vi "Feedback 3 (SubVI).vi"(0 "reset_in":bool, 1 "eta_dot_last":dbl[](array[numeric]), 5 "Nu":dbl[](array[numeric]), 7 "Eta_last":dbl[](array[numeric]), 9 "Wait criteria":dbl[](array[numeric])=[2.0, 2.0, 2.0, 0.1], 11 "Restart criteria":dbl[](array[numeric])=[0.5, 0.5, 0.5, 0.1], 12 "Eta":dbl[](array[numeric]), 13 "Eta_d":dbl[](array[numeric]), 14 "Eta_ref":dbl[](array[numeric])) -> (4 "Boolean":bool, 6 "reset":bool, 8 "Eta_ref_out":dbl[](array[numeric]), 10 "u0":dbl[](array[numeric]), 15 "x0_out":dbl[](array[numeric]))   [LabVIEW 2011]
uses:
  <vilib>/imath/engines/lvmath2/RunTimeEngine/ErrorHandling/NIMS_Finalize Error.vi
  <vilib>/imath/engines/lvmath2/RunTimeEngine/Managers/WorkSpace/UID Generator.vi
  <vilib>/imath/engines/lvmath2/RunTimeEngine/RangeToken/NIMS_Range_R2 - Integer.vi
  <instcachedir>/0/NIMS_Range_R2 - Integer_8B99B1FAA0BB43C693F13B8216F464EC.lvgen/NIMS_Range_R2 - Integer_8B99B1FAA0BB43C693F13B8216F464EC_000.vi
  <vilib>/imath/engines/lvmath2/RunTimeEngine/Managers/SymbolTable/Clear UID.vi
  <vilib>/imath/engines/lvmath2/RunTimeEngine/NodeEndStatement/NIMS_NodeEndStatement_Output.vi
  <instcachedir>/0/NIMS_NodeEndStatement_Output_53EC0D466D134D7ABD903AC30B43404B.lvgen/NIMS_NodeEndStatement_Output_53EC0D466D134D7ABD903AC30B43404B_005.vi
  <vilib>/imath/engines/lvmath2/RunTimeEngine/CommandStatement/MC_CommandStatement_break.vi
  <vilib>/imath/engines/lvmath2/RunTimeEngine/VariableToken/Read/NIMS_Get Elements - RV(_) - Check.vi
  <instcachedir>/0/NIMS_Get Elements - RV(_) - Check_B511B9D8E05044FE80F9F088FE24B20C.lvgen/NIMS_Get Elements - RV(_) - Check_B511B9D8E05044FE80F9F088FE24B20C_000.vi
  <vilib>/imath/engines/lvmath2/RunTimeEngine/ErrorHandling/NIMS_Create Error From Enums.vi
  <vilib>/imath/engines/lvmath2/RunTimeEngine/ReplaceToken/NIMS_Replace - Check Linear.vi
  <instcachedir>/0/NIMS_Replace - Check Linear_276AD648BD064726893CCF9ED6E2A728.lvgen/NIMS_Replace - Check Linear_276AD648BD064726893CCF9ED6E2A728_001.vi
  <vilib>/imath/engines/lvmath2/RunTimeEngine/ReplaceToken/NIMS_Replace - Size Check _(_)=S.vi
  <instcachedir>/0/NIMS_Replace - Size Check _(_)=S_9ABE7AF2D26C43EAA05192D5C1E6C624.lvgen/NIMS_Replace - Size Check _(_)=S_9ABE7AF2D26C43EAA05192D5C1E6C624_000.vi
  <vilib>/imath/engines/lvmath2/RunTimeEngine/ReplaceToken/NIMS_Replace - V(S)=S.vi
  <instcachedir>/0/NIMS_Replace - V(S)=S_16B13A4565AB46F59881314645612498.lvgen/NIMS_Replace - V(S)=S_16B13A4565AB46F59881314645612498_000.vi
  <vilib>/imath/engines/lvmath2/RunTimeEngine/RunTimeType/NIMS_RunTimeType_From StrictType (excl LVString).vi
  <instcachedir>/0/NIMS_RunTimeType_From StrictType (excl LVString)_46AE8B54A11948F0BCCEB8091EE7AA4C.lvgen/NIMS_RunTimeType_From StrictType (excl LVString)_46AE8B54A11948F0BCCEB8091EE7AA4C_000.vi
  <vilib>/imath/engines/lvmath2/RunTimeEngine/LocalVariableDefStatement/MC_LocalVariableDefStatement_Display.vi
  <vilib>/imath/engines/lvmath2/RunTimeEngine/NodeEndStatement/NIMS_NodeEndStatement_Get Vector.vi
  <instcachedir>/0/NIMS_NodeEndStatement_Get Vector_50E2F48DC826428EA11CD85545CBACBE.lvgen/NIMS_NodeEndStatement_Get Vector_50E2F48DC826428EA11CD85545CBACBE_003.vi
  <instcachedir>/0/NIMS_NodeEndStatement_Get Vector_50E2F48DC826428EA11CD85545CBACBE.lvgen/NIMS_NodeEndStatement_Get Vector_50E2F48DC826428EA11CD85545CBACBE_001.vi
  <vilib>/imath/engines/lvmath/Functions/Error Handling/MergeErrorsWrapper.vi
  <instcachedir>/0/NIMS_NodeEndStatement_Output_53EC0D466D134D7ABD903AC30B43404B.lvgen/NIMS_NodeEndStatement_Output_53EC0D466D134D7ABD903AC30B43404B_013.vi
  <instcachedir>/0/NIMS_NodeEndStatement_Output_53EC0D466D134D7ABD903AC30B43404B.lvgen/NIMS_NodeEndStatement_Output_53EC0D466D134D7ABD903AC30B43404B_012.vi
  <instcachedir>/0/NIMS_NodeEndStatement_Output_53EC0D466D134D7ABD903AC30B43404B.lvgen/NIMS_NodeEndStatement_Output_53EC0D466D134D7ABD903AC30B43404B_001.vi
  <vilib>/imath/engines/lvmath2/RunTimeEngine/VariableToken/Read/NIMS_Get Elements - SorM(_) - Check.vi
  <instcachedir>/0/NIMS_Get Elements - SorM(_) - Check_6C920A4996D9400D8D9F035318A663F0.lvgen/NIMS_Get Elements - SorM(_) - Check_6C920A4996D9400D8D9F035318A663F0_007.vi
  <vilib>/imathl/engines/lvmath/Functions/Error Handling/Create Error.vi
  <instcachedir>/0/NIMS_Replace - Check Linear_276AD648BD064726893CCF9ED6E2A728.lvgen/NIMS_Replace - Check Linear_276AD648BD064726893CCF9ED6E2A728_006.vi
  <instcachedir>/0/NIMS_Replace - Size Check _(_)=S_9ABE7AF2D26C43EAA05192D5C1E6C624.lvgen/NIMS_Replace - Size Check _(_)=S_9ABE7AF2D26C43EAA05192D5C1E6C624_004.vi
  <vilib>/imath/engines/lvmath2/RunTimeEngine/ReplaceToken/NIMS_Replace - M(S)=S.vi
  <instcachedir>/0/NIMS_Replace - M(S)=S_FF4DE4724B384A588EB88F1DEAD450CF.lvgen/NIMS_Replace - M(S)=S_FF4DE4724B384A588EB88F1DEAD450CF_001.vi
  <vilib>/imath/engines/lvmath2/RunTimeEngine/ArithmeticOperatorToken/NIMS_ArithmeticOperator_multmx(M,CV).vi
  <instcachedir>/0/NIMS_ArithmeticOperator_multmx(M,CV)_B95E4EDD04E247939487CF1FF34819AA.lvgen/NIMS_ArithmeticOperator_multmx(M,CV)_B95E4EDD04E247939487CF1FF34819AA_000.vi
  <vilib>/imath/engines/lvmath2/RunTimeEngine/BuiltInFunctions/abs/NIMS_abs(signed).vi
  <instcachedir>/0/NIMS_abs(signed)_C4FCB8E6058B49B797C7C8D53CA5F6EC.lvgen/NIMS_abs(signed)_C4FCB8E6058B49B797C7C8D53CA5F6EC_000.vi
  <instcachedir>/0/NIMS_Get Elements - SorM(_) - Check_6C920A4996D9400D8D9F035318A663F0.lvgen/NIMS_Get Elements - SorM(_) - Check_6C920A4996D9400D8D9F035318A663F0_000.vi
  <vilib>/imath/engines/lvmath2/RunTimeEngine/ArithmeticOperatorToken/NIMS_ArithmeticOperator_minus.vi
  <instcachedir>/0/NIMS_ArithmeticOperator_minus_27860A2576AF4B729B9D72749D8AAD88.lvgen/NIMS_ArithmeticOperator_minus_27860A2576AF4B729B9D72749D8AAD88_003.vi
  <vilib>/imath/engines/lvmath2/RunTimeEngine/Managers/SymbolTable/NIMS_WorkSpace.lvlib
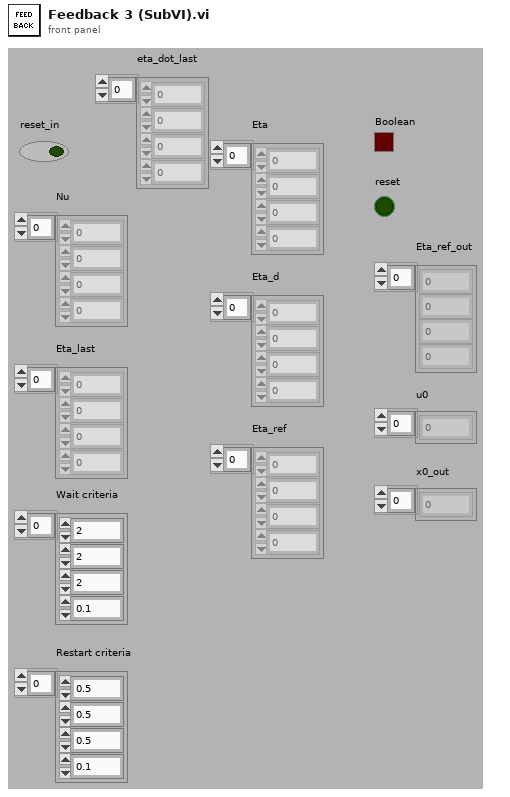
[diagram p1: front panel]
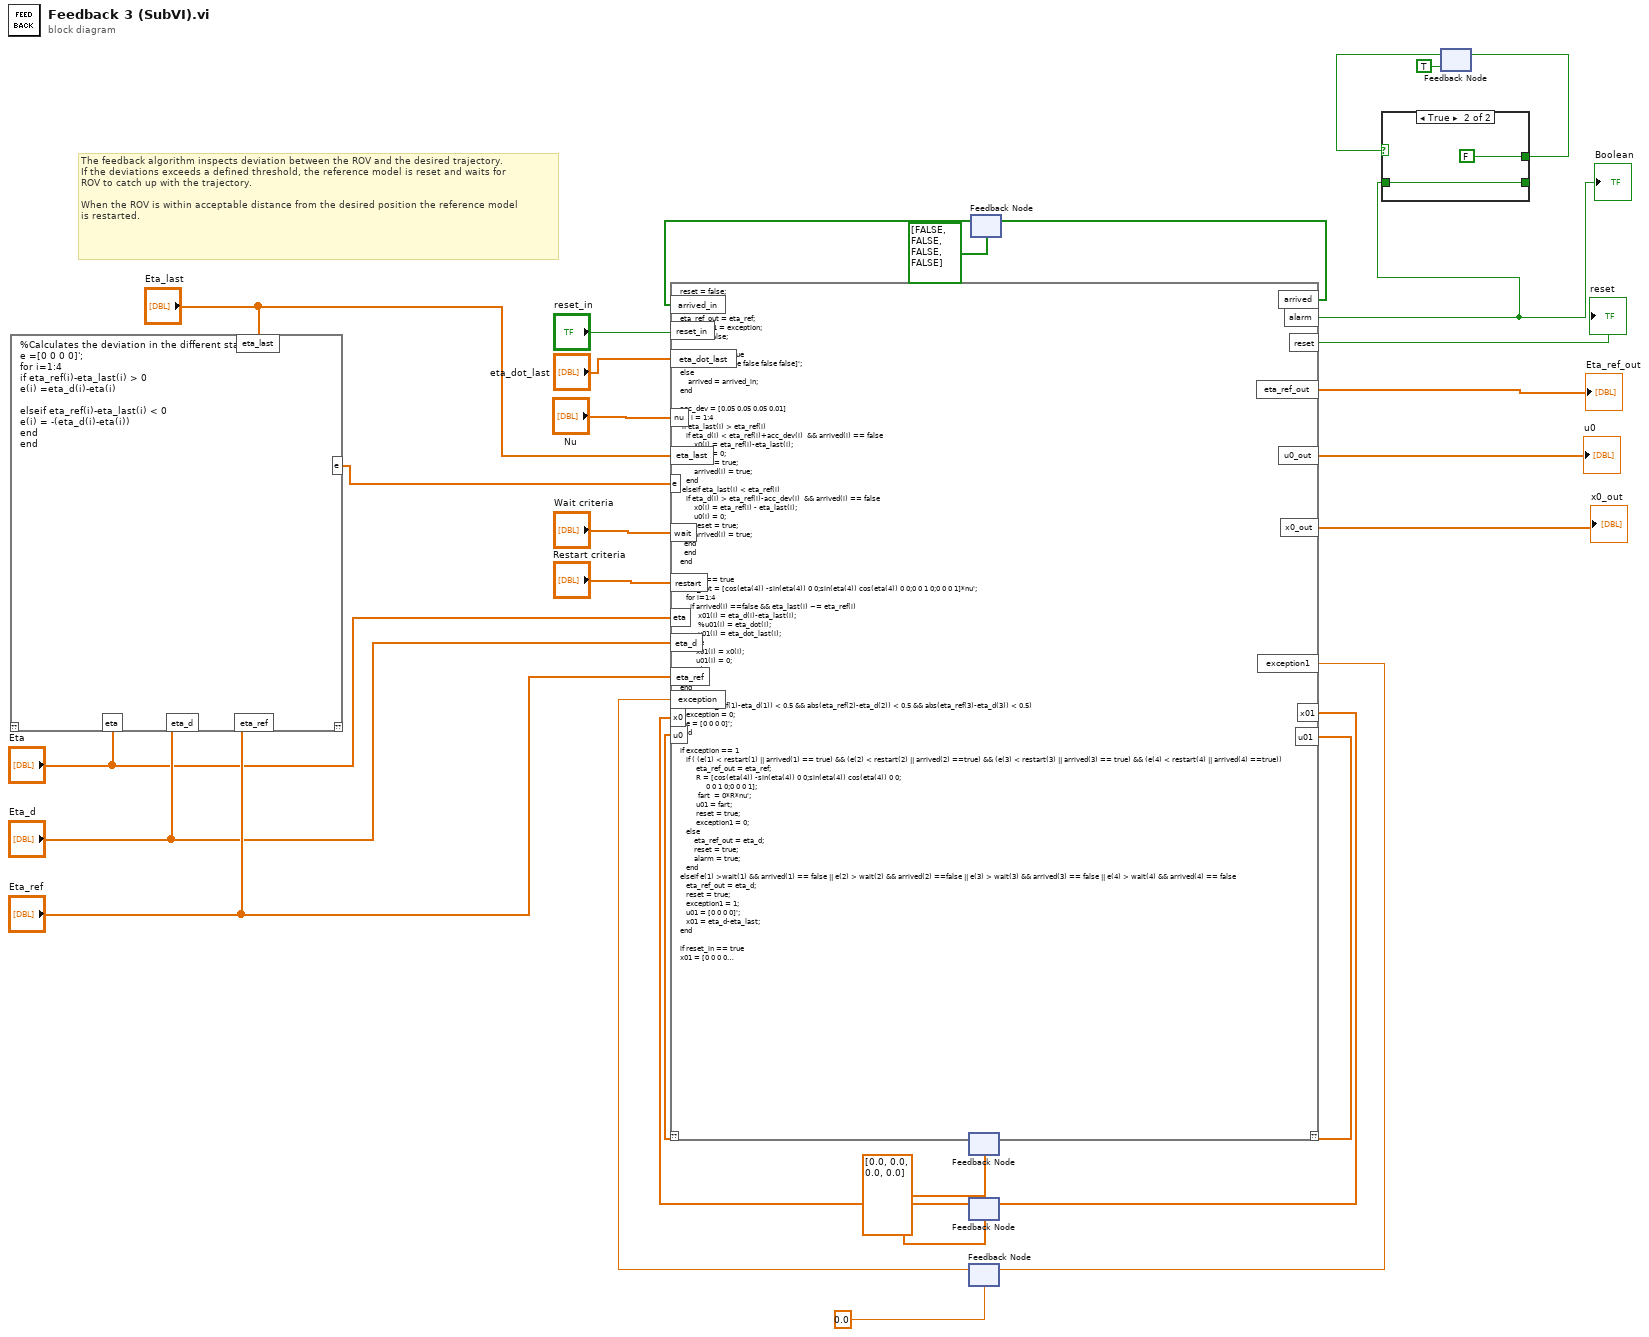
[diagram p0: block diagram]
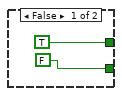
[diagram p2: hidden frame]
diagram:
  w23 = dbl[] [0.0, 0.0, 0.0, 0.0]
  # "The feedback algorithm inspects deviation between the ROV and the desired trajectory.\nIf the deviations exceeds a defined threshold, the reference model is reset and waits for\nROV to catch up with the trajectory. \n\nWhen the ROV is within acceptable distance from the desired position the reference model\nis restarted."
  n1 = mathscript code="%Calculates the deviation in the different states.\ne =[0 0 0 0]';\nfor i=1:4\nif eta_ref(i)-eta_last(i) > 0 \ne(i) =eta_d(i)-eta(i)\n\nelseif eta_ref(i)-eta_last(i) < 0\ne(i) = -(eta_d(i)-eta(i))\nend\nend"("eta_last"="Eta_last", "eta"="Eta", "eta_d"="Eta_d", "eta_ref"="Eta_ref") -> ("e"=w22:dbl[])  [unwired: 1 in, 1 out]
  n2 = feedback #1(w23) -> (w16:dbl[])
  n3 = feedback #2(w23) -> (w6:dbl[])
  n4 = feedback #3(0.0) -> (w14:dbl)
  n5 = feedback #4(bool[] [FALSE, FALSE, FALSE, FALSE]) -> (w3:bool[])
  n6 = mathscript code="reset = false;\nu01 = u0;\nx01 = x0;\neta_ref_out = eta_ref; \nexception1 = exception;\nalarm = false;\n\nif reset_in == true\n    arrived = [false false false false]';\nelse\n    arrived = arrived_in;\nend\n\nacc_dev = [0.05 0.05 0.05 0.01]\nfor i = 1:4\n if eta_last(i) > eta_ref(i)   \n   if eta_d(i) < eta_ref(i)+acc_dev(i)  && arrived(i) == false\n       x0(i) = eta_ref(i)-eta_last(i);\n       u0(i) = 0; \n       reset = true; \n       arrived(i) = true;\n   end \n elseif eta_last(i) < eta_ref(i) \n   if eta_d(i) > eta_ref(i)-acc_dev(i)  && arrived(i) == false\n       x0(i) = eta_ref(i) - eta_last(i);\n       u0(i) = 0;\n       reset = true;\n       arrived(i) = true;\n  end\n  end\nend\n\nif reset == true\n   eta_dot = [cos(eta(4)) -sin(eta(4)) 0 0;sin(eta(4)) cos(eta(4)) 0 0;0 0 1 0;0 0 0 1]*nu';\n   for i=1:4\n     if arrived(i) ==false && eta_last(i) ~= eta_ref(i)\n         x01(i) = eta_d(i)-eta_last(i);\n         %u01(i) = eta_dot(i);\n         u01(i) = eta_dot_last(i);\n     else\n        x01(i) = x0(i);\n        u01(i) = 0;\n     end\n   end\nend\n\nif (abs(eta_ref(1)-eta_d(1)) < 0.5 && abs(eta_ref(2)-eta_d(2)) < 0.5 && abs(eta_ref(3)-eta_d(3)) < 0.5)\n   exception = 0;\n   e = [0 0 0 0]';\nend\n\nif exception == 1\n   if ( (e(1) < restart(1) || arrived(1) == true) && (e(2) < restart(2) || arrived(2) ==true) && (e(3) < restart(3) || arrived(3) == true) && (e(4) < restart(4) || arrived(4) ==true))\n        eta_ref_out = eta_ref;\n        R = [cos(eta(4)) -sin(eta(4)) 0 0;sin(eta(4)) cos(eta(4)) 0 0;\n             0 0 1 0;0 0 0 1];\n         fart  = 0*R*nu';\n        u01 = fart; \n        reset = true;\n        exception1 = 0;\n   else\n       eta_ref_out = eta_d;\n       reset = true;\n       alarm = true;\n   end\nelseif e(1) >wait(1) && arrived(1) == false || e(2) > wait(2) && arrived(2) ==false || e(3) > wait(3) && arrived(3) == false || e(4) > wait(4) && arrived(4) == false\n   eta_ref_out = eta_d;\n   reset = true;\n   exception1 = 1;\n   u01 = [0 0 0 0]';\n   x01 = eta_d-eta_last;\nend\n\nif reset_in == true\nx01 = [0 0 0 0]';\nu01 = [0 0 0 0]';\neta_ref_out = eta_ref;\nexception = 0;\nreset = true;\nend\n\nx0_out = x01;\nu0_out = u01;"("e"=w22, "eta_d"="Eta_d", "exception"=w14, "eta_ref"="Eta_ref", "nu"="Nu", "eta"="Eta", "u0"=w16, "reset_in"="reset_in", "x0"=w6, "eta_last"="Eta_last", "wait"="Wait criteria", "restart"="Restart criteria", "arrived_in"=w3, "eta_dot_last"="eta_dot_last") -> ("exception1"=w15:dbl, "eta_ref_out"=→"Eta_ref_out":dbl[], "u01"=w11:dbl[], "u0_out"=→"u0":dbl[], "reset"=→"reset":bool, "x01"=w7:dbl[], "x0_out"=→"x0_out":dbl[], "alarm"=w29:bool, "arrived"=w4:bool[])  [unwired: 1 in, 1 out]
  "Boolean" <- w29
  n7 = feedback-in #1(w11) -> ()
  n8 = feedback-in #2(w7) -> ()
  n9 = feedback-in #3(w15) -> ()
  n10 = feedback-in #4(w4) -> ()
  n11 = feedback #5(TRUE) -> (w27:bool)
  n12 = case shown="True" w27 {
    tunnel: [TRUE FALSE] -> w26
    tunnel: w29 -> [_ w32]
    tunnel: [FALSE w32] -> _
    frame False {
    }
    frame True {
    }
  }
  n13 = feedback-in #5(w26) -> ()
